vi "Write_IntakeCommand.vi"(8 "error in (no error)":errorcluster, 10 "Intake Command":T1, 11 "IntakeData in":refnum<class "IntakeData.lvclass">) -> (0 "error out":errorcluster, 3 "IntakeData out":refnum<class "IntakeData.lvclass">)   [LabVIEW 2017, in "IntakeData.lvclass"]
uses:
  IntakeData.lvclass
  Team-code/IntakeCommand.ctl
  IntakeData.lvclass/IntakeData.ctl
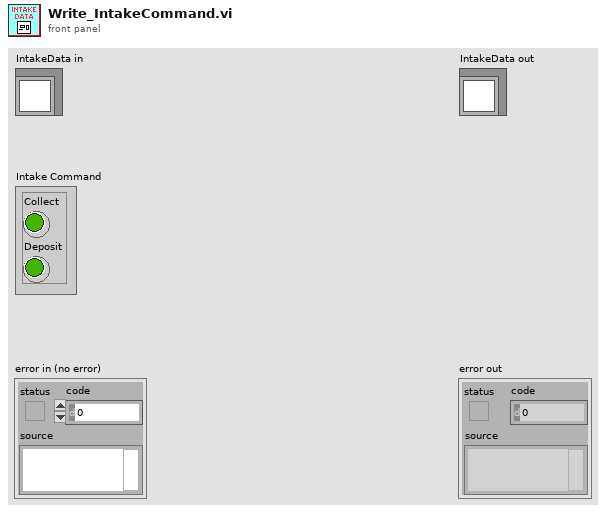
[diagram p1: front panel]
types:
  T1 = typedef "IntakeData.lvclass/IntakeCommand.ctl" = cluster{"Collect":bool, "Deposit":bool}
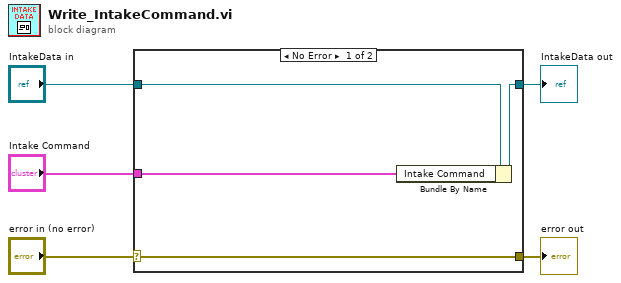
[diagram p0: block diagram]
diagram:
  n1 = case shown="No Error" "error in (no error)" {
    selector: "error in (no error)" -> [w9 w10]
    tunnel: [w9 w10] -> w4
    tunnel: [w7 w11] -> w2
    tunnel: "IntakeData in" -> [w8 w11]
    tunnel: "Intake Command" -> [w6 _]
    frame No Error {
      n2 = Bundle By Name(cluster=w8, "Intake Command"=w6) -> (w7:refnum<class "IntakeData.lvclass">)
    }
    frame Error {
    }
  }
  "error out" <- w4
  "IntakeData out" <- w2
